vi "Area Scoring.vi"(10 "Convex Hull Area":dbl, 11 "Area":dbl) -> (3 "Score":dbl)   [LabVIEW 2014]
doc: "Calculate a score based on area and convex hull area. Convex hull area fills holes and convex areas of the shape. It is equivalent to putting a rubbed band around the shape and computing the area of the band."
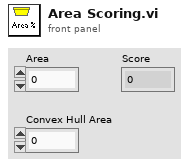
[diagram p1: front panel]
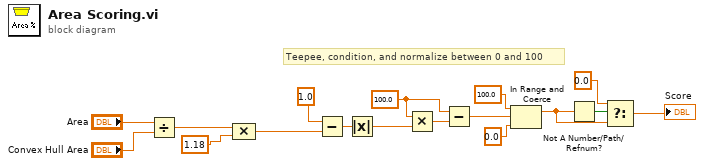
[diagram p0: block diagram]
diagram:
  w8 = 100.0 ("x/y")
  # "Teepee, condition, and normalize between 0 and 100"
  n1 = Divide(x="Area", y="Convex Hull Area") -> (x/y=w15:dbl)
  n2 = Compound Arithmetic op=MULTIPLY(w15, 1.18 ("length")) -> (w2:dbl)
  n3 = Subtract(x=1.0 ("y"), y=w2) -> (x-y=w6:dbl)
  n4 = Absolute Value(x=w6) -> (abs(x)=w9:dbl)
  n5 = Multiply(x=w8, y=w9) -> (x*y=w10:dbl)
  n6 = Subtract(x=w8, y=w10) -> (x-y=w5:dbl)
  n7 = In Range and Coerce(upper limit=100.0, x=w5, lower limit=0.0) -> (coerced(x)=w13:dbl)  [unwired: 1 out]
  n8 = Not A Number/Path/Refnum?(number/path/refnum=w13) -> (NaN/Path/Refnum?=w12:bool)
  n9 = Select(t=0.0 ("y"), s=w12, f=w13) -> (s? t:f=→"Score":dbl)
